vi "Hope This Works.vi"() -> ()   [LabVIEW 2018]
uses:
  <vilib>/vision/NI_Vision_Development_Module.lvlib
panel:
  in  "Foaia de citit":path=path "D:/Work/Sesiune Stiintifica 2019/Labview/Alphabet.jpg"
  in  "Alfabetul":path=path "D:/Work/Sesiune Stiintifica 2019/Labview/alphabet space oops end.abc"
  out "Read String":string
  in  "Rectangle":T1 {"Rotation" min=-90.0 max=90.0 step=1.0 format="%.2f"; "Left" scale=0.0..1024.0; "Right" scale=0.0..1024.0}
  out "Image":T2(plugin-control)
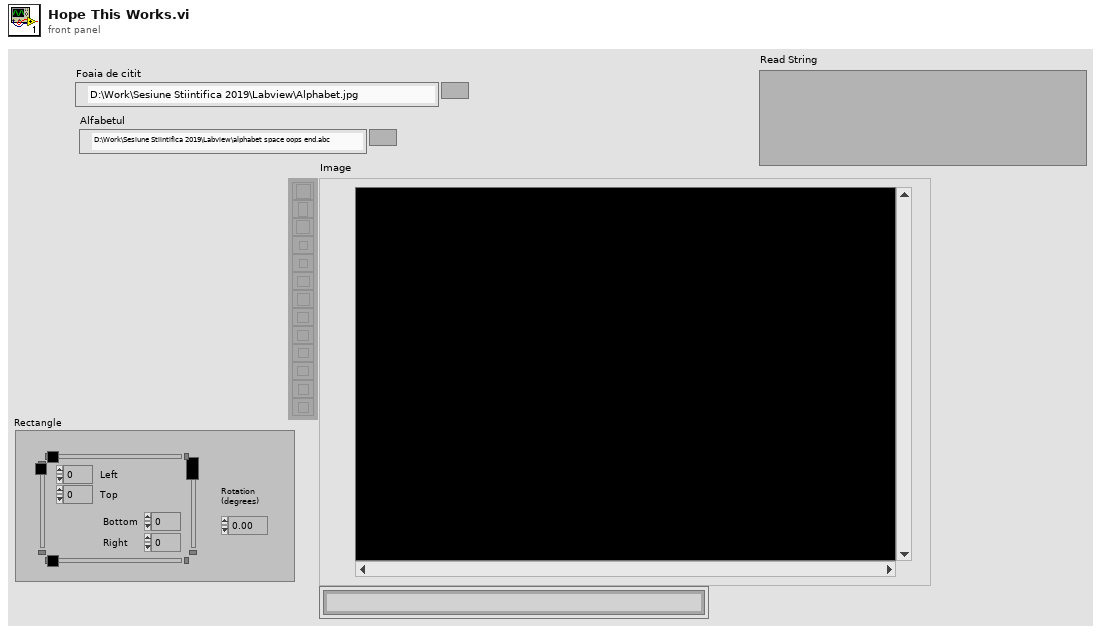
[diagram p1: front panel]
types:
  T1 = typedef "IMAQ Rectangle" = cluster{"Left":i32, "Top":i32, "Right":i32, "Bottom":i32, "Rotation":dbl}
  T2 = typedef "IMAQ Image.ctl" = refnum<image>
  T3 = typedef "IMAQ OCR Session.ctl" = refnum<k1>
  T4 = typedef "ROI Descriptor" = cluster{"Global Rectangle":i32[], "Contours":cluster{"ID":enum32{"External", "Internal"}, "Type":u32, "Coordinates":i32[]}[]}
  T5 = cluster{"Global Rectangle":i32[], "Contours":cluster{"ID":enum32{"External", "Internal"}, "Type":u32, "Coordinates":i32[]}[]}
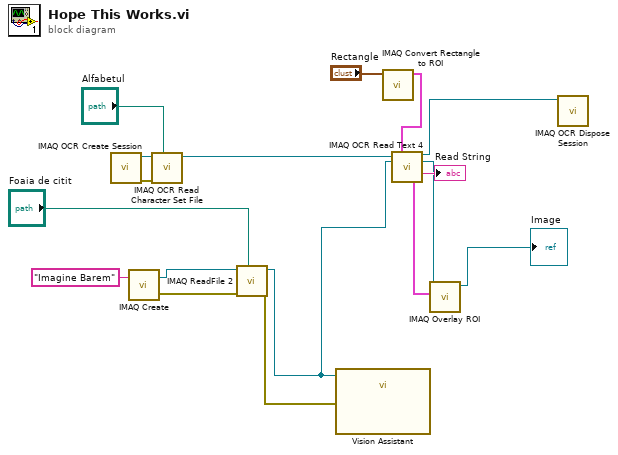
[diagram p0: block diagram]
diagram:
  n1 = call "IMAQ OCR Create Session"() -> ("error out"=w11:errorcluster, "IMAQ OCR Session"=w12:T3)  [unwired: 10 in]
  n2 = call "IMAQ Create"("Image Name"="Imagine Barem") -> ("New Image"=w16:T2, "error out"=w14:errorcluster)  [unwired: 4 in]
  n3 = call "IMAQ OCR Read Character Set File"("File Path"="Alfabetul", "error in (no error)"=w11, "IMAQ OCR Session"=w12) -> ("IMAQ OCR Session (dup)"=w2:T3)  [unwired: 6 in, 2 out]
  n4 = call "IMAQ ReadFile 2"("File Path"="Foaia de citit", "error in (no error)"=w14, "Image"=w16) -> ("error out"=w13:errorcluster, "Image Out"=w3:T2)  [unwired: 4 in, 3 out]
  n5 = call "Vision Assistant"("Image In"=w3, "error in"=w13) -> ()  [unwired: 24 in, 2 out]
  n6 = call "IMAQ Convert Rectangle to ROI"("Rectangle"="Rectangle") -> ("ROI Descriptor"=w8:T4)  [unwired: 8 in, 1 out]
  n7 = call "IMAQ OCR Read Text 4"("IMAQ OCR Session"=w2, "ROI Descriptor"=w8, "Image"=w3) -> ("IMAQ OCR Session (dup)"=w1:T3, "Image (dup)"=w6:T2, "Read String"=→"Read String":string, "ROI Bounding Characters"=w5:T5)  [unwired: 6 in, 3 out]
  n8 = call "IMAQ Overlay ROI"("ROI Descriptor"=w5, "Image"=w6) -> ("Image Out"=→"Image":T2)  [unwired: 8 in, 1 out]
  n9 = call "IMAQ OCR Dispose Session"("IMAQ OCR Session"=w1) -> ()  [unwired: 10 in, 1 out]
